vi "Bracket Balancing.VI"(1 "string before":string) -> (0 "string after":string)   [LabVIEW 2014, in "NI_Gmath.lvlib"]
uses:
  NI_Gmath.lvlib
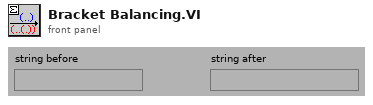
[diagram p1: front panel]
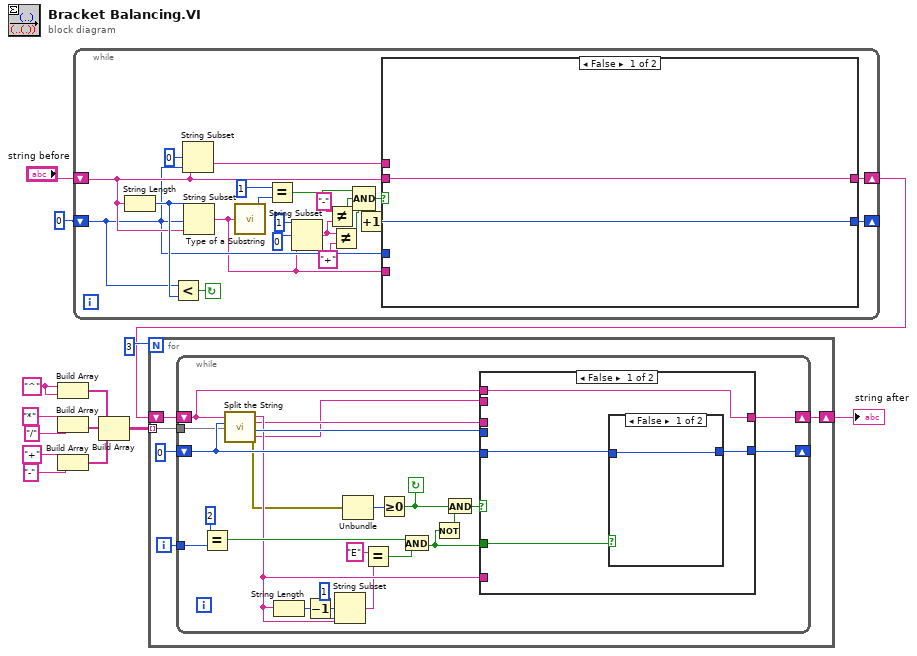
[diagram p0: block diagram]
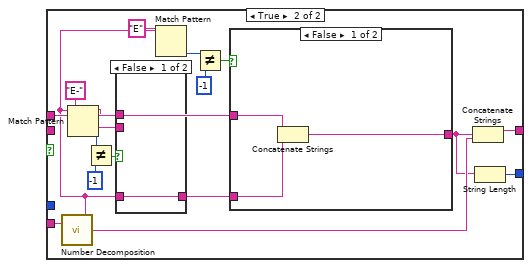
[diagram p2: hidden frame]
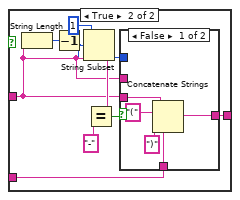
[diagram p3: hidden frame]
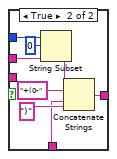
[diagram p4: hidden frame]
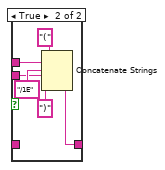
[diagram p5: hidden frame]
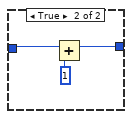
[diagram p6: hidden frame]
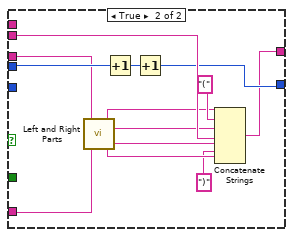
[diagram p7: hidden frame]
diagram:
  w5 = "^"
  n1 = Build Array(w5, w5) -> (w9:string[])
  n2 = Build Array("*", "/") -> (w8:string[])
  n3 = Build Array("+", "-") -> (w7:string[])
  n4 = while {
    shift-left: "string before" -> [w28]
    shift-right: [w25] -> w1
    shift-left: 0 -> [w26]
    shift-right: [w31] -> _
    stop <- w29 continue-if-true
    n5 = String Length(string=w28) -> (length=w30:i32)
    n6 = Less?(x=w26, y=w30) -> (x < y?=w29:bool)
    n7 = String Subset(string=w28, offset (0)=0, length (rest)=w26) -> (substring=w27:string)
    n8 = String Subset(string=w28, offset (0)=w26, length (rest)=w30) -> (substring=w24:string)
    n9 = call "Type of a Substring.VI"("item"=w24) -> ("type"=w32:i32)
    n10 = Equal?(x=1, y=w32) -> (x = y?=w20:bool)
    n11 = String Subset(string=w24, offset (0)=0, length (rest)=1) -> (substring=w19:string)
    n12 = Not Equal?(x="-", y=w19) -> (x != y?=w17:bool)
    n13 = Not Equal?(x=w19, y="+") -> (x != y?=w18:bool)
    n14 = Compound Arithmetic op=AND(w20, w17, w18) -> (w21:bool)
    n15 = case shown="False" w21 {
      tunnel: w26 -> [w37 _]
      tunnel: [w36 w51] -> w31
      tunnel: w28 -> [w35 _]
      tunnel: [w35 w53] -> w25
      tunnel: w24 -> [_ w55]
      tunnel: w27 -> [_ w50]
      frame False {
        n16 = Increment(x=w37) -> (x+1=w36:i32)
      }
      frame True {
        n17 = call "Number Decomposition.VI"("number string"=w55) -> ("number"=w42:string, "rest"=w54:string)  [unwired: 1 in, 1 out]
        n18 = Match Pattern(string=w42, regular expression="E-") -> (before substring=w48:string, after substring=w49:string, offset past match=w45:i32)  [unwired: 1 in, 1 out]
        n19 = Not Equal?(x=w45, y=-1) -> (x != y?=w47:bool)
        n20 = case shown="False" w47 {
          tunnel: w42 -> [w81 _]
          tunnel: [w81 w83] -> w43
          tunnel: w48 -> [_ w86]
          tunnel: w49 -> [_ w84]
          frame False {
          }
          frame True {
            n21 = Concatenate Strings("(", w86, "/1E", w84, ")") -> (w83:string)
          }
        }
        n22 = Match Pattern(string=w42, regular expression="E") -> (offset past match=w40:i32)  [unwired: 1 in, 3 out]
        n23 = Not Equal?(x=w40, y=-1) -> (x != y?=w39:bool)
        n24 = case shown="False" w39 {
          tunnel: w43 -> [w56 w67]
          tunnel: w50 -> [w58 w60]
          tunnel: [w57 w62] -> w52
          frame False {
            n25 = Concatenate Strings(w58, w56) -> (w57:string)
          }
          frame True {
            n26 = String Length(string=w60) -> (length=w66:i32)
            n27 = Decrement(x=w66) -> (x-1=w59:i32)
            n28 = String Subset(string=w60, offset (0)=w59, length (rest)=1) -> (substring=w61:string)
            n29 = Equal?(x=w61, y="-") -> (x = y?=w63:bool)
            n30 = case shown="False" w63 {
              tunnel: w60 -> [w72 _]
              tunnel: [w71 w80] -> w62
              tunnel: w67 -> [w68 w77]
              tunnel: w60 -> [_ w76]
              tunnel: w59 -> [_ w74]
              frame False {
                n31 = Concatenate Strings(w72, "(", w68, ")") -> (w71:string)
              }
              frame True {
                n32 = String Subset(string=w76, offset (0)=0, length (rest)=w74) -> (substring=w73:string)
                n33 = Concatenate Strings(w73, "+(0-", w77, ")") -> (w80:string)
              }
            }
          }
        }
        n34 = Concatenate Strings(w52, w54) -> (w53:string)
        n35 = String Length(string=w52) -> (length=w51:i32)
      }
    }
  }
  n36 = Build Array(w9, w8, w7) -> (w13:string[][])
  n37 = for {
    N: 3 -> [_]
    shift-right: [w88] -> w2
    shift-left: w1 -> [w91]
    tunnel: w13 -> [w92] mode=indexing
    i -> [w89]
    n38 = while {
      tunnel: w89 -> [w115]
      tunnel: w92 -> [w100]
      shift-left: 0 -> [w106]
      shift-right: [w116] -> _
      shift-left: w91 -> [w99]
      shift-right: [w95] -> w88
      stop <- w96 continue-if-true
      n39 = Equal?(x=2, y=w115) -> (x = y?=w109:bool)
      n40 = call "Split the String.vi"("Marker"=w100, "position"=w106, "string"=w99) -> ("error out"=w102:errorcluster, "choice"=w103:string, "new position"=w107:i32, "after"=w104:string, "before"=w105:string)  [unwired: 1 in]
      n41 = String Length(string=w105) -> (length=w113:i32)
      n42 = Decrement(x=w113) -> (x-1=w112:i32)
      n43 = String Subset(string=w105, offset (0)=w112, length (rest)=1) -> (substring=w94:string)
      n44 = Unbundle(w102) -> ("code"=w101:i32)  [unwired: 2 out]
      n45 = Equal?(x="E", y=w94) -> (x = y?=w110:bool)
      n46 = Greater Or Equal To 0?(x=w101) -> (x >= 0?=w96:bool)
      n47 = And(x=w109, y=w110) -> (x .and. y?=w97:bool)
      n48 = Not(x=w97) -> (.not. x?=w108:bool)
      n49 = And(x=w96, y=w108) -> (x .and. y?=w98:bool)
      n50 = case shown="False" w98 {
        tunnel: w104 -> [_ w129]
        tunnel: w105 -> [_ w125]
        tunnel: [w120 w126] -> w95
        tunnel: w103 -> [_ w136]
        tunnel: [w117 w131] -> w116
        tunnel: w106 -> [w118 _]
        tunnel: w99 -> [w120 _]
        tunnel: w107 -> [_ w130]
        tunnel: w97 -> [w119 _]
        frame False {
          n51 = case shown="False" w119 {
            tunnel: w118 -> [w121 w124]
            tunnel: [w121 w122] -> w117
            frame False {
            }
            frame True {
              n52 = Add(x=w124, y=1) -> (x+y=w122:i32)
            }
          }
        }
        frame True {
          n53 = call "Left and Right Parts.vi"("after"=w129, "before"=w125) -> ("left start"=w127:string, "left end"=w128:string, "right start"=w133:string, "right end"=w135:string)
          n54 = Increment(x=w130) -> (x+1=w137:i32)
          n55 = Increment(x=w137) -> (x+1=w131:i32)
          n56 = Concatenate Strings(w127, "(", w128, w136, w133, ")", w135) -> (w126:string)
        }
      }
    }
  }
  "string after" <- w2
